vi "Configure_Interrupt_Threshold.vi"(7 "I2C Channel":u8, 8 "error in":errorcluster, 9 "Interrupt Threshold":u8, 10 "Interrupt Source":T1(ring), 11 "LINX Resource In":T2) -> (0 "error out":errorcluster, 2 "Full-Scale Adjusted Threshold":dbl, 3 "LINX Resource Out":T2)   [LabVIEW 2014, in "LMH-LINX.lvlib" / "LIS331HH.lvlib"]
uses:
  <vilib>/MakerHub/LINX/Public/Sensors/Accelerometer/LIS331HH/LIS331HH.lvlib
  <vilib>/MakerHub/LINX/Private/Type Defs/LINX Ref.ctl
  <vilib>/MakerHub/LINX/Private/Type Defs/Platform.ctl
  <vilib>/MakerHub/LINX/Private/Type Defs/Interface.ctl
  <vilib>/MakerHub/LINX/Private/Device/Type Defs/LINX Device Config.ctl
  <vilib>/MakerHub/LINX/Private/Device/Type Defs/TCP Config.ctl
  <vilib>/MakerHub/LINX/Private/Device/Type Defs/Channels.ctl
  <vilib>/MakerHub/LINX/Private/Local IO/LinxI2cWrite.vi
  <vilib>/MakerHub/LINX/Public/Utilities/Check Channel.vi
  <vilib>/MakerHub/LINX/Private/Utilties/Generate Error.vi
  <vilib>/MakerHub/LINX/LMH-LINX.lvlib
  <vilib>/MakerHub/LINX/Private/Device/Device.lvlib
panel:
  # "INPUTS"
  # "OUTPUTS"
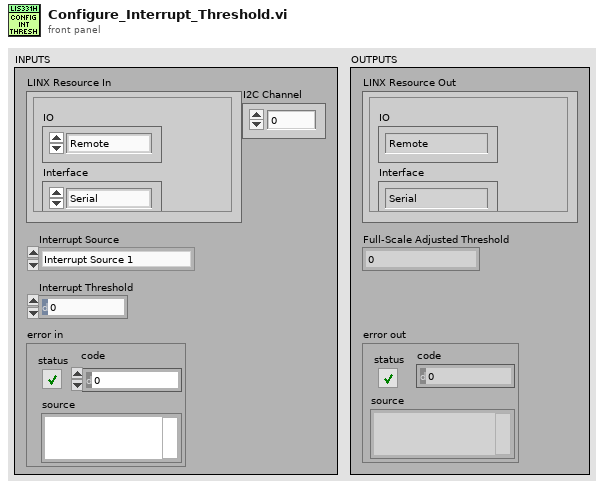
[diagram p1: front panel]
types:
  T1 = enum16{"Interrupt Source 1", "Interrupt Source 2"}
  T2 = typedef "LMH-LINX.lvlib/LINX Ref.ctl" = cluster{"IO":T3, "Interface":T4, "LINX Device Config":T5}
  T3 = typedef "LMH-LINX.lvlib/Platform.ctl" = enum16{"Remote", "Local"}
  T4 = typedef "LMH-LINX.lvlib/Interface.ctl" = enum16{"Serial", "TCP"}
  T5 = typedef "LMH-LINX.lvlib/Device.lvlib/LINX Device Config.ctl" = cluster{"Interface":T4, "COM Port":refnum<visa-resource-name>, "TCP Configuration":T6, "Device Family":u8, "Device ID":u8, "Device Name":string, "TCP Ref":refnum<k5>, "Channels":T7}
  T6 = typedef "LMH-LINX.lvlib/Device.lvlib/TCP Config.ctl" = cluster{"IP Address":string, "Port":u16}
  T7 = typedef "LMH-LINX.lvlib/Channels.ctl" = cluster{"DI":u8[], "DO":u8[], "AI":u8[], "AO":u8[], "PWM":u8[], "QE":u8[], "UART":u8[], "I2C 2":u8[], "SPI":u8[], "CAN":u8[], "Servo":u8[], "AI Ref (V)":dbl, "AI Resolution (Bits)":u8, "AO Ref (V)":dbl, "AO Resolution (Bits)":u8}
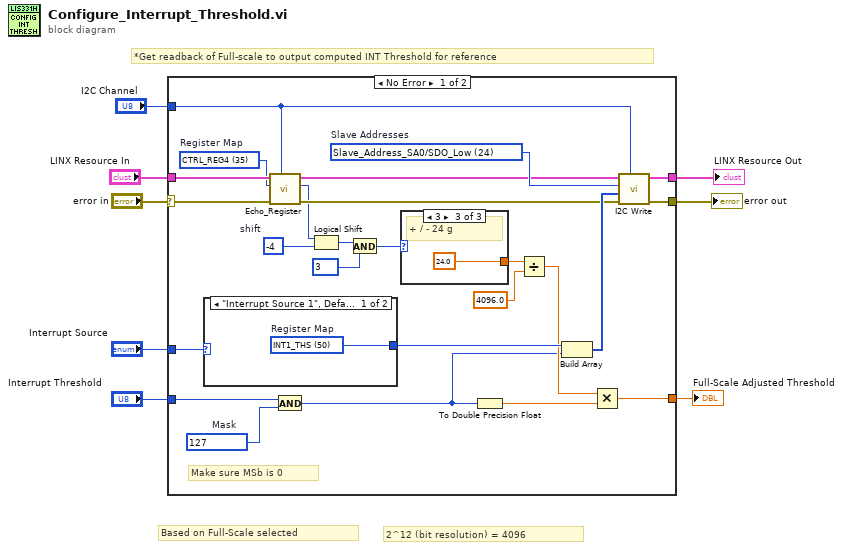
[diagram p0: block diagram]
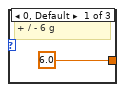
[diagram p2: hidden frame]
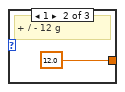
[diagram p3: hidden frame]
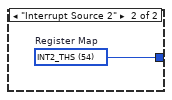
[diagram p4: hidden frame]
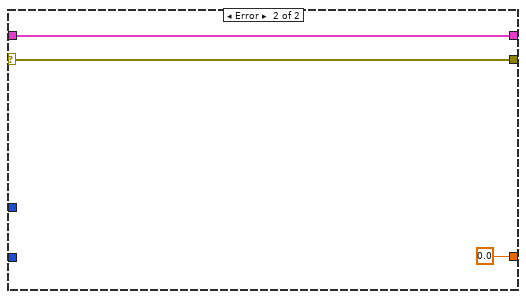
[diagram p5: hidden frame]
diagram:
  # "2^12 (bit resolution) = 4096"
  # "*Get readback of Full-scale to output computed INT Threshold for reference"
  # "Based on Full-Scale selected"
  n1 = case shown="No Error" "error in" {
    selector: "error in" -> [w24 w41]
    tunnel: [w32 w41] -> w7
    tunnel: "LINX Resource In" -> [w25 w40]
    tunnel: "I2C Channel" -> [w21 _]
    tunnel: [w33 w40] -> w4
    tunnel: "Interrupt Source" -> [w30 _]
    tunnel: "Interrupt Threshold" -> [w27 _]
    tunnel: [w12 0.0] -> w1
    frame No Error {
      w18 = i8 -4  # shift
      w20 = u8 35 items=["CTRL_REG1"=32, "CTRL_REG2"=33, "CTRL_REG3"=34, "CTRL_REG4"=35, "CTRL_REG5"=36, "HP_FILTER_RESET"=37, "REFERENCE"=38, "STATUS_REG"=39, "OUT_X_L"=40, "OUT_X_H"=41, "OUT_Y_L"=42, "OUT_Y_H"=43, "OUT_Z_L"=44, "OUT_Z_H"=45, "INT1_CFG"=48, "INT1_SOURCE"=49, "INT1_THS"=50, "INT1_DURATION"=51, "INT2_CFG"=52, "INT2_SOURCE"=53, "INT2_THS"=54, "INT2_DURATION"=55]  # Register Map
      w26 = u8 127  # Mask
      w31 = u8 24 items=["Slave_Address_SA0/SDO_Low"=24, "Slave_Address_SA0/SDO_High"=25]  # Slave Addresses
      # "Make sure MSb is 0"
      n2 = case shown="\"Interrupt Source 1\", Default" w30 {
        tunnel: [w37 w38] -> w29
        frame "Interrupt Source 1", Default {
          w37 = u8 50 items=["CTRL_REG1"=32, "CTRL_REG2"=33, "CTRL_REG3"=34, "CTRL_REG4"=35, "CTRL_REG5"=36, "HP_FILTER_RESET"=37, "REFERENCE"=38, "STATUS_REG"=39, "OUT_X_L"=40, "OUT_X_H"=41, "OUT_Y_L"=42, "OUT_Y_H"=43, "OUT_Z_L"=44, "OUT_Z_H"=45, "INT1_CFG"=48, "INT1_SOURCE"=49, "INT1_THS"=50, "INT1_DURATION"=51, "INT2_CFG"=52, "INT2_SOURCE"=53, "INT2_THS"=54, "INT2_DURATION"=55]  # Register Map
        }
        frame "Interrupt Source 2" {
          w38 = u8 54 items=["CTRL_REG1"=32, "CTRL_REG2"=33, "CTRL_REG3"=34, "CTRL_REG4"=35, "CTRL_REG5"=36, "HP_FILTER_RESET"=37, "REFERENCE"=38, "STATUS_REG"=39, "OUT_X_L"=40, "OUT_X_H"=41, "OUT_Y_L"=42, "OUT_Y_H"=43, "OUT_Z_L"=44, "OUT_Z_H"=45, "INT1_CFG"=48, "INT1_SOURCE"=49, "INT1_THS"=50, "INT1_DURATION"=51, "INT2_CFG"=52, "INT2_SOURCE"=53, "INT2_THS"=54, "INT2_DURATION"=55]  # Register Map
        }
      }
      n3 = call <vilib>:"Echo_Register.vi"("I2C Channel"=w21, "error in (no error)"=w24, "Register to Echo"=w20, "LINX Resource In"=w25) -> ("error out"=w23:errorcluster, "Register Word"=w19:u8, "LINX Resource Out"=w22:T2)  [unwired: 5 in]
      n4 = And(x=w27, y=w26) -> (x .and. y?=w14:u8)
      n5 = Logical Shift(y=w19, x=w18) -> (x << y=w11:i8)
      n6 = And(x=w11, y=i8 3) -> (x .and. y?=w10:i8)
      n7 = case shown="3" w10 {
        tunnel: [6.0 12.0 24.0] -> w17
        frame 0, Default {
          # "+ / - 6 g"
        }
        frame 1 {
          # "+ / - 12 g"
        }
        frame 3 {
          # "+ / - 24 g"
        }
      }
      n8 = To Double Precision Float(number=w14) -> (double precision float=w13:dbl)
      n9 = Divide(x=w17, y=4096.0) -> (x/y=w15:dbl)
      n10 = Build Array(w29, w14) -> (w28:u8[])
      n11 = Multiply(x=w15, y=w13) -> (x*y=w12:dbl)
      n12 = call <vilib>:"I2C Write.vi"("I2C Channel"=w21, "Error In"=w23, "Data"=w28, "I2C Slave Address (0)"=w31, "LINX Resource"=w22) -> ("Error Out"=w32:errorcluster, "LINX Resource"=w33:T2)  [unwired: 5 in]
    }
    frame Error {
    }
  }
  "error out" <- w7
  "LINX Resource Out" <- w4
  "Full-Scale Adjusted Threshold" <- w1
